vi "Increment Group Iteration.vi"(8 "error in (no error)":errorcluster, 11 "Transfer Group Timing in":refnum<class "Transfer Group Timing.lvclass">) -> (0 "error out":errorcluster, 3 "Transfer Group Timing out":refnum<class "Transfer Group Timing.lvclass">)   [LabVIEW 2017, in "DSF Core.lvlib" / "Transfer Group Timing.lvclass"]
uses:
  Transfer Group Timing.lvclass
  Transfer Group Timing.lvclass/Transfer Group Timing.ctl
  Timing.lvclass/Timing.ctl
  Timing.lvclass
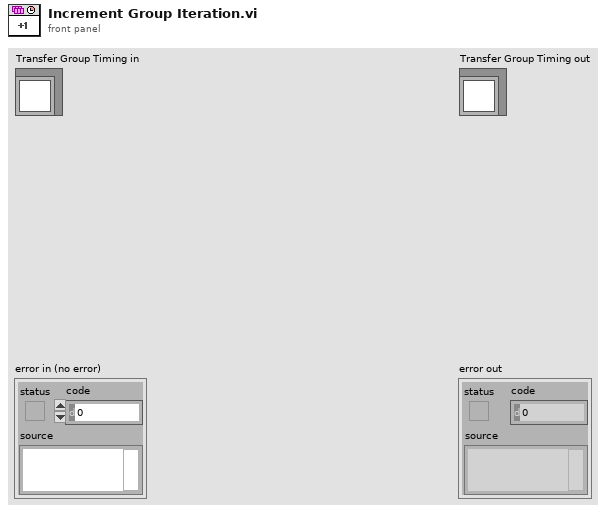
[diagram p1: front panel]
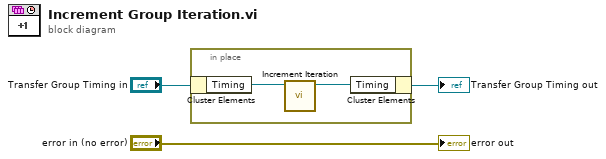
[diagram p0: block diagram]
diagram:
  n1 = in-place {
    n2 = in-place-cluster #1("Transfer Group Timing in") -> ("Timing"=w5:refnum<class "Timing.lvclass">)
    n3 = call "Increment Iteration.vi"("Timing in"=w5) -> ("Timing out"=w4:refnum<class "Timing.lvclass">)  [unwired: 10 in]
    n4 = in-place-cluster #1("Timing"=w4) -> (→"Transfer Group Timing out":refnum<class "Transfer Group Timing.lvclass">)
  }
  "error out" <- "error in (no error)"
